vi "Process.vi"(11 "Message Queues out":T1) -> ()   [LabVIEW 2024]
doc: "This UI handle all the data process including data acquisition and calculations"
uses:
  Message Queue/All Message Queues.ctl
  Message Queue/Message Cluster.ctl
  controls/GlobalData.ctl
  controls/GlobalData.vi
  Message Queue/Enqueue Message (Single).vi
  Message Queue/Message Queue.lvlib
panel:
  out "Acquire Time":u32
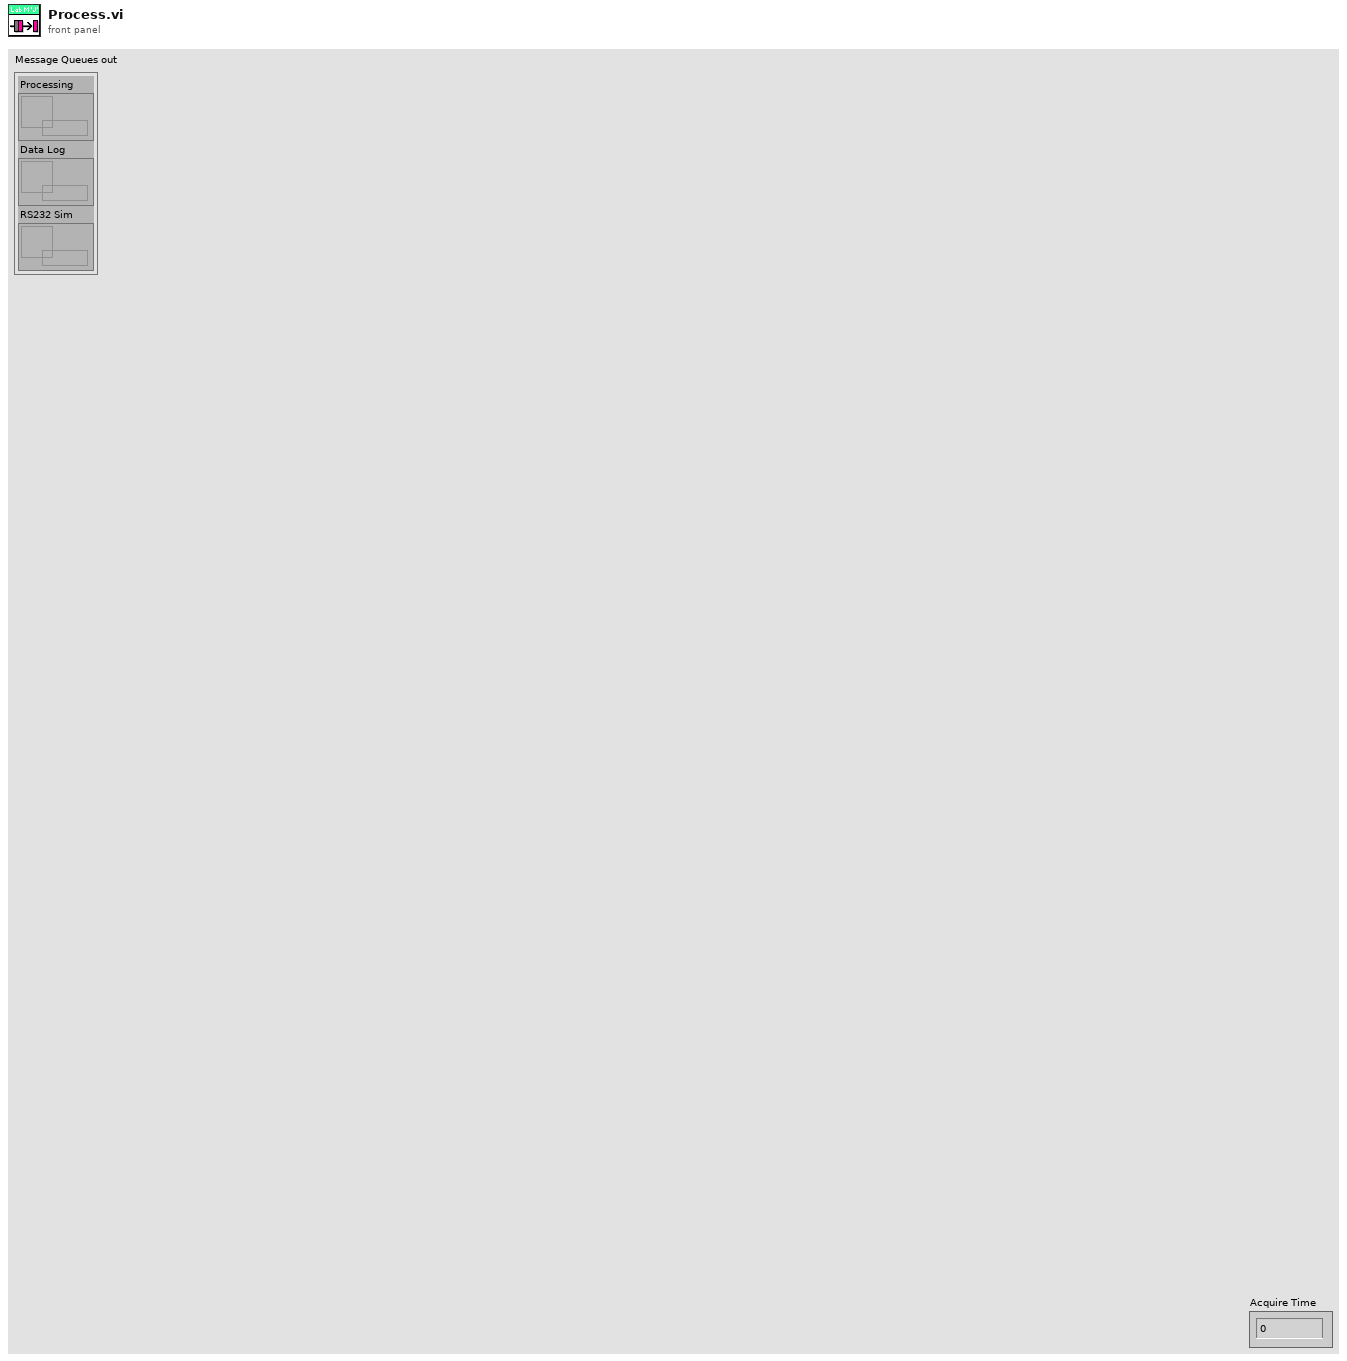
[diagram p1: front panel]
types:
  T1 = typedef "Message Queue.lvlib/All Message Queues.ctl" = cluster{"Processing":refnum<queue>, "Data Log":refnum<queue>, "RS232 Sim":refnum<queue>}
  T2 = typedef "GlobalData.ctl" = cluster{"Measurements":cluster{"Measurement Graphs":refnum<vi>, "Pressure":refnum<vi>, "Temperature":refnum<vi>, "Salinity":refnum<vi>, "Weight":refnum<vi>, "Pressure Raw":refnum<vi>, "Temperature Raw":refnum<vi>, "Salinity Raw":refnum<vi>, "Weight Raw":refnum<vi>, "Measurement Statstics":refnum<vi>, "Time Array":refnum<vi>}, "Settings":cluster{"Sampling Settings":refnum<vi>, "General Settings":refnum<vi>, "Disable Sensor Reading":refnum<vi>, "Units Settings":refnum<vi>, "Channels Settings":refnum<vi>, "Weight Port Settings":refnum<vi>}, "Calibration Data":cluster{"Pressure Cal":refnum<vi>, "Temperature Cal":refnum<vi>, "Salinity Cal":refnum<vi>, "Weight Cal":refnum<vi>}, "UI":cluster{"Generate Report":refnum<vi>}}
  T3 = cluster{"Pressure":dbl[], "Temperature":dbl[], "Salinity":dbl[], "Weight":dbl[]}
  T4 = cluster{"Measurement Statstics":bool, "Logging Type":enum16{"Disable Log", "TDMS", "CSV"}}
  T5 = cluster{"Reading Time (ms)":u64, "Graph Time ":u16}
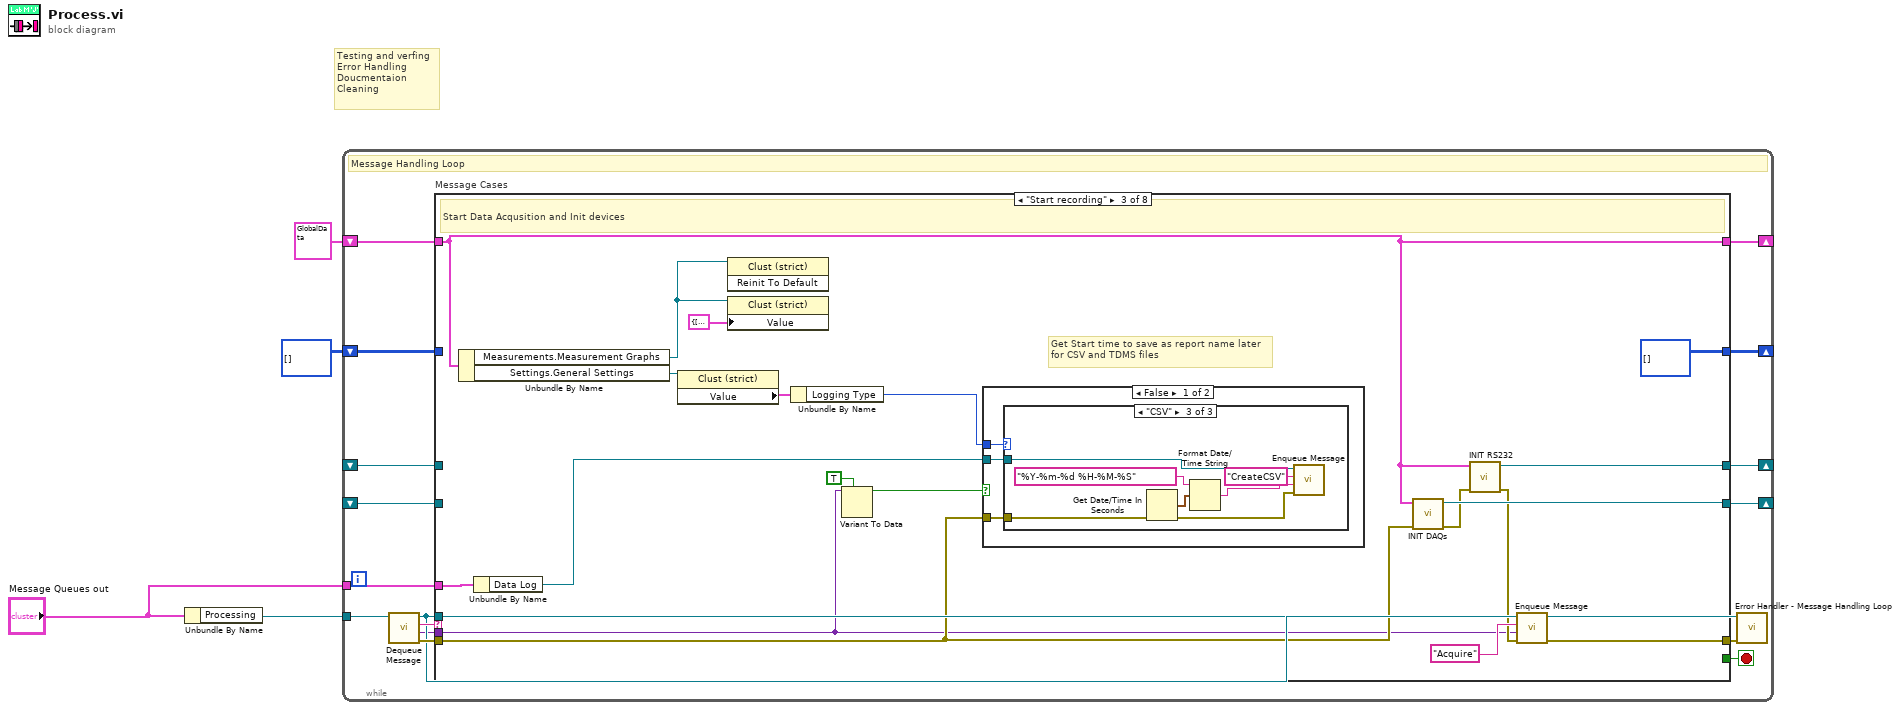
[diagram p0: block diagram]
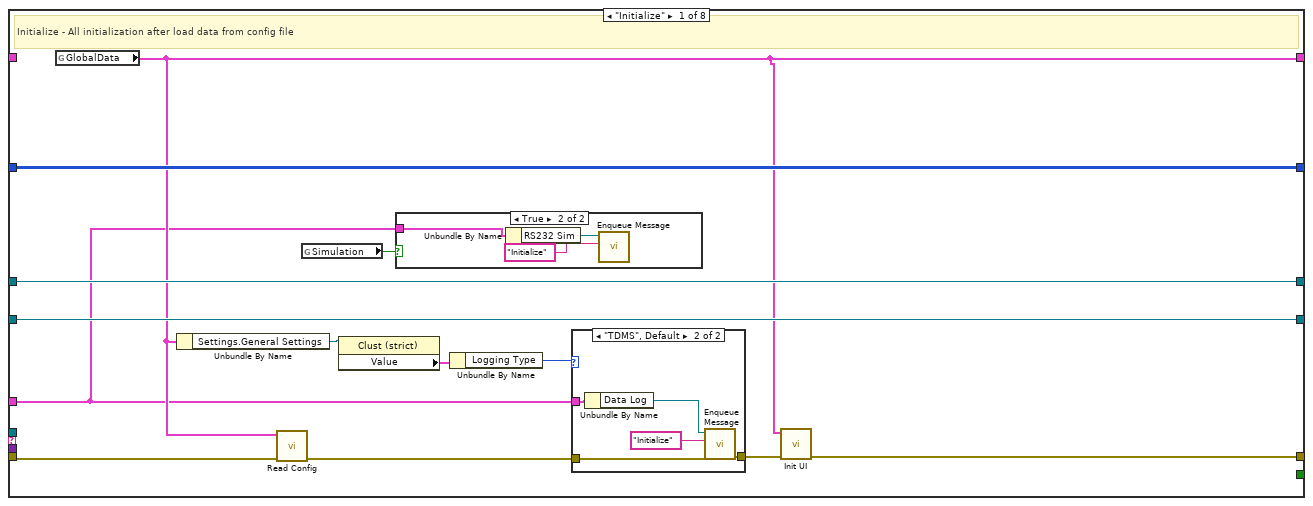
[diagram p2: hidden frame]
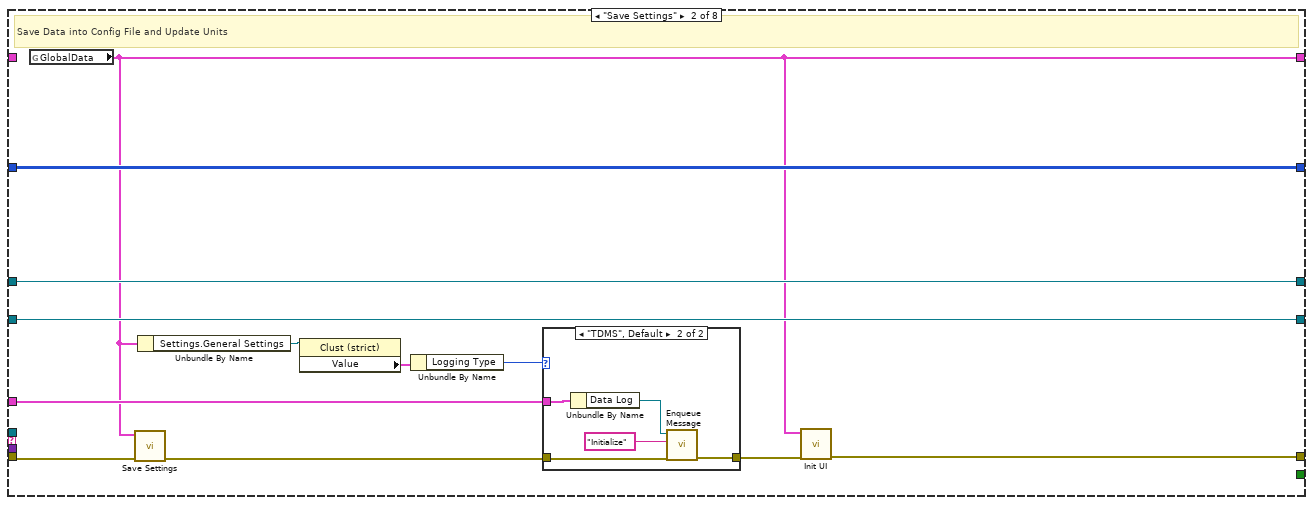
[diagram p5: hidden frame]
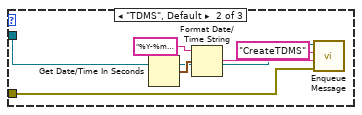
[diagram p8: hidden frame]
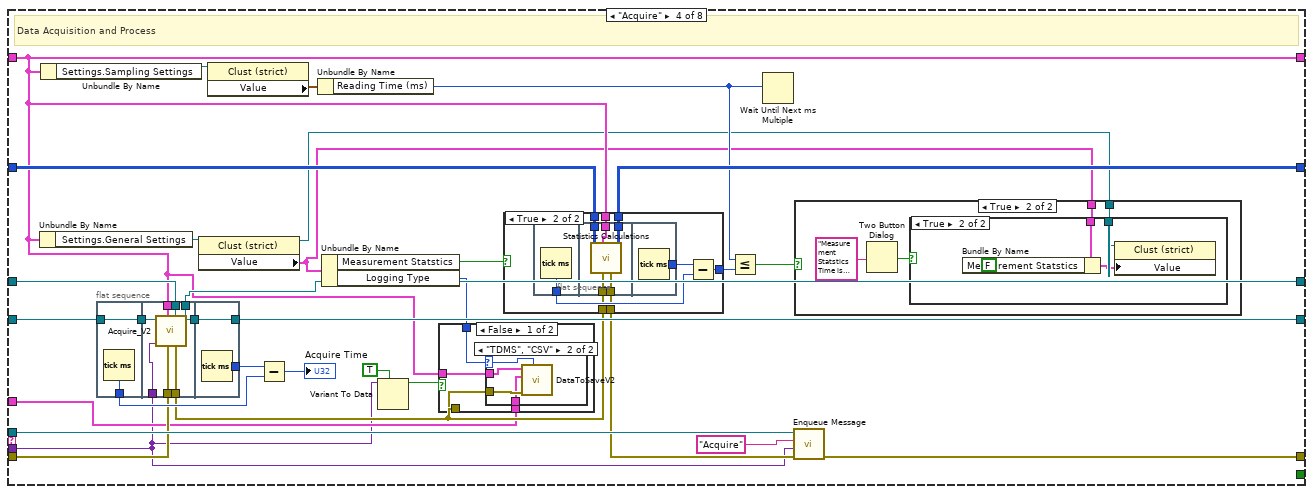
[diagram p10: hidden frame]
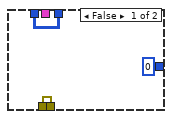
[diagram p15: hidden frame]
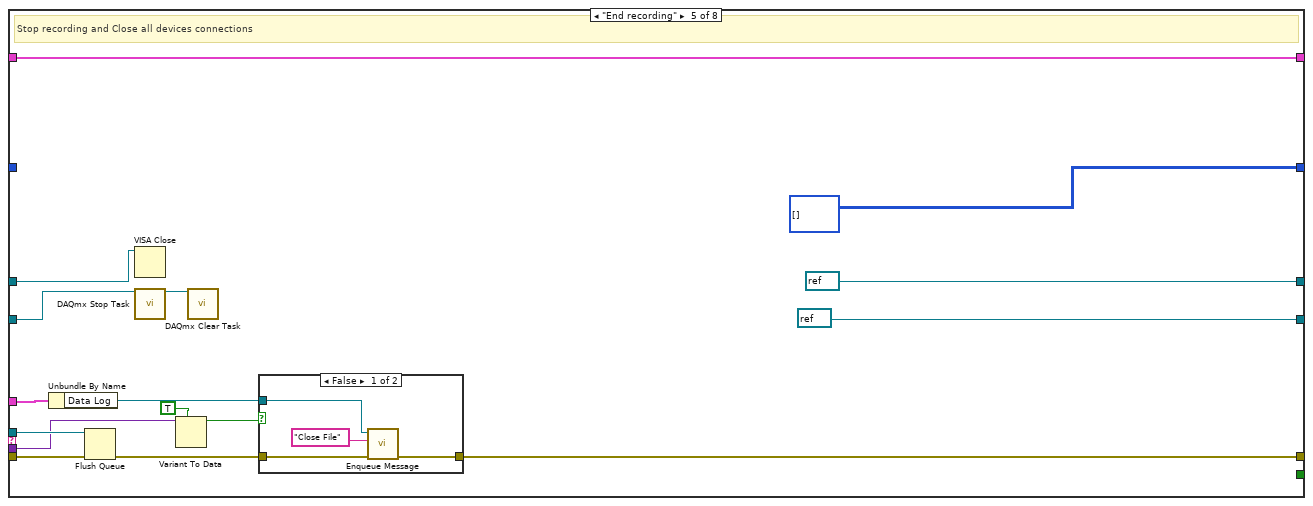
[diagram p16: hidden frame]
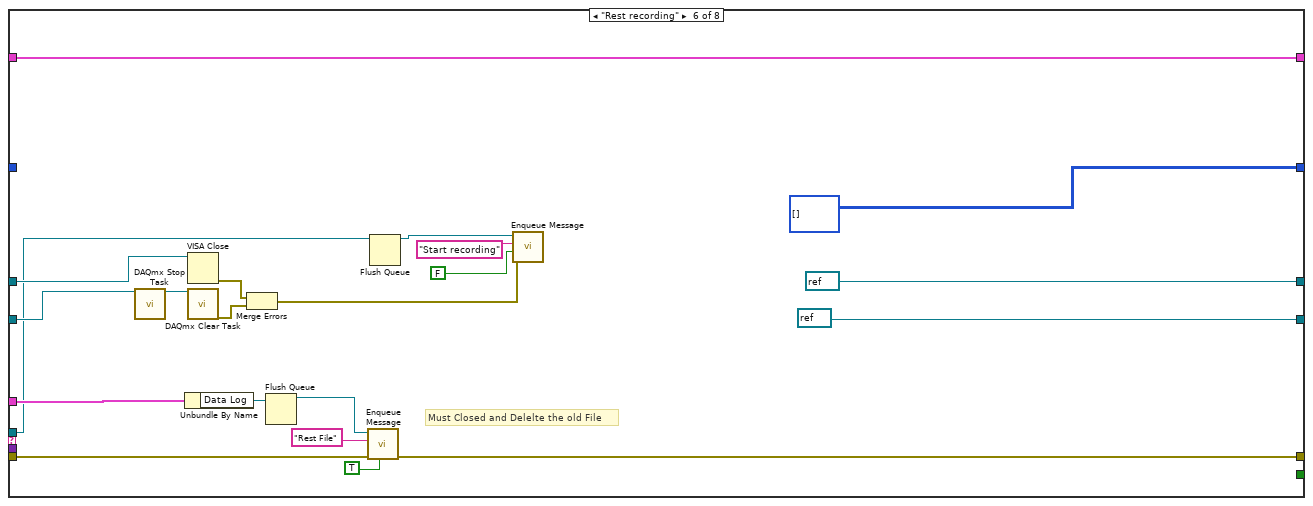
[diagram p18: hidden frame]
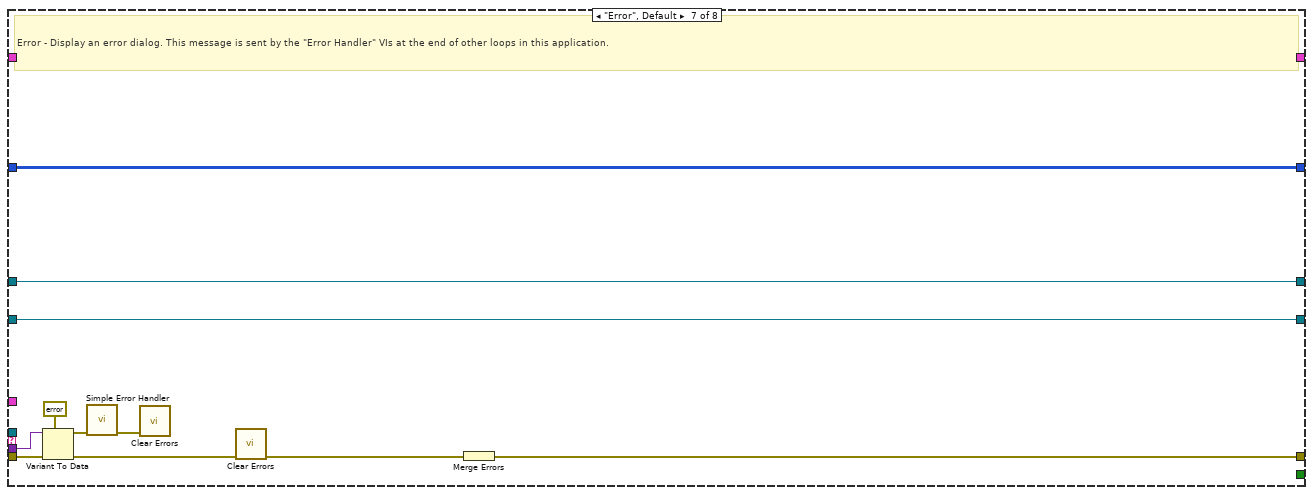
[diagram p19: hidden frame]
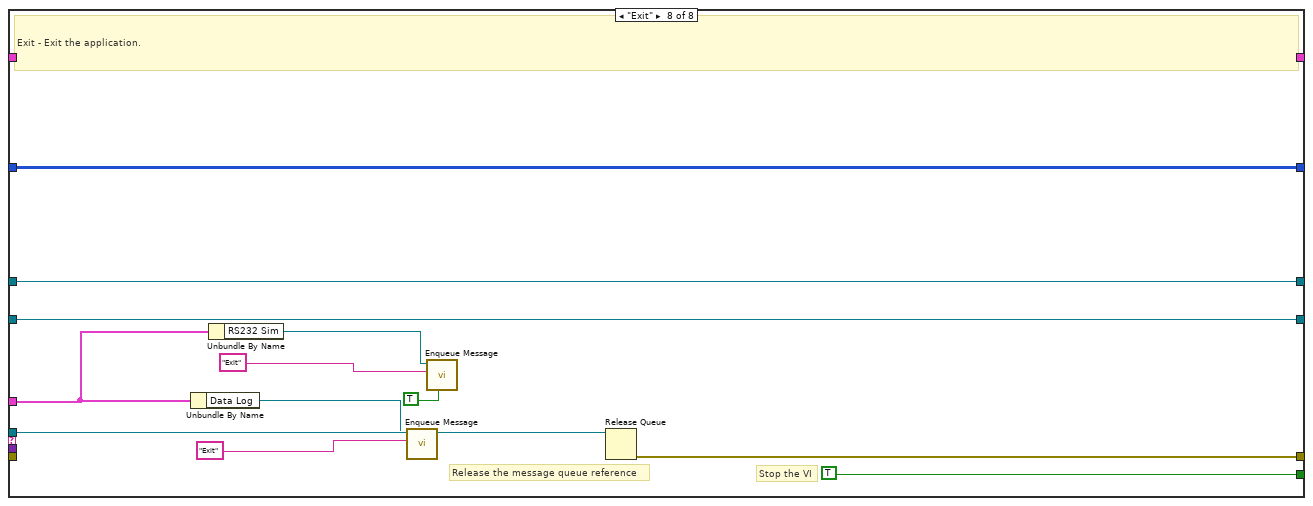
[diagram p20: hidden frame]
diagram:
  # "Testing and verfing\nError Handling \nDoucmentaion\nCleaning"
  n1 = Unbundle By Name("Message Queues out") -> ("Processing"=w4:refnum<queue>)
  n2 = while {
    tunnel: w4 -> [w15]
    shift-right: [w19] -> _
    shift-left: T2 {"Measurements"={"Measurement Graphs"=refnum, "Pressure"=refnum, "Temperature"=refnum, "Salinity"=refnum, "Weight"=refnum, "Pressure Raw"=refnum, "Temperature Raw"=refnum, "Salinity Raw"=refnum, "Weight Raw"=refnum, "Measurement Statstics"=refnum, "Time Array"=refnum}, "Settings"={"Sampling Settings"=refnum, "General Settings"=refnum, "Disable Sensor Reading"=refnum, "Units Settings"=refnum, "Channels Settings"=refnum, "Weight Port Settings"=refnum}, "Calibration Data"={"Pressure Cal"=refnum, "Temperature Cal"=refnum, "Salinity Cal"=refnum, "Weight Cal"=refnum}, "UI"={"Generate Report"=refnum}} ("GlobalData") -> [w20]
    shift-right: [w12] -> _
    shift-left: _ -> [w11]
    shift-right: [w9] -> _
    shift-left: i32[][] [] -> [w10]
    shift-right: [w7] -> _
    shift-left: _ -> [w6]
    tunnel: "Message Queues out" -> [w5]
    stop <- w18 stop-if-true
    # "Message Handling Loop"
    n3 = call "Dequeue Message.vi"("Message Queue"=w15) -> ("error out"=w17:errorcluster, "Message Data"=w8:variant, "Message"=w16:string, "dup Message Queue"=w14:refnum<queue>)  [unwired: 7 in]
    n4 = case "Message Cases" shown="\"Start recording\"" w16 {
      tunnel: w14 -> [_ _ w76 w124 w179 w204 _ w239]
      tunnel: w17 -> [w29 w49 w69 w105 w181 w206 w226 _]
      tunnel: [w30 w51 w78 w123 w180 w205 w221 w231] -> w13
      tunnel: w20 -> [_ _ w64 w102 w188 w214 w225 w238]
      tunnel: [w26 w44 w64 w102 w188 w214 w225 w238] -> w19
      tunnel: [_ _ _ _ _ _ _ TRUE] -> w18
      tunnel: [w33 w54 w80 w126 refnum<k21> refnum ("Pressure") refnum<k21> refnum ("Pressure") w220 w236] -> w12
      tunnel: w11 -> [w33 w54 _ w127 w186 w212 w220 w236]
      tunnel: w10 -> [w32 w53 _ w116 _ _ w219 w235]
      tunnel: [w32 w53 i32[][] [] ("Time Array") w115 i32[][] [] ("Time Array") i32[][] [] ("Time Array") w219 w235] -> w9
      tunnel: w8 -> [_ _ w62 w98 w174 _ w224 _]
      tunnel: [w31 w52 w74 w106 refnum<visa-resource-name> refnum ("Weight Port") refnum<visa-resource-name> refnum ("Weight Port") w218 w234] -> w7
      tunnel: w6 -> [w31 w52 _ w107 w184 w210 w218 w234]
      tunnel: w5 -> [w21 w50 w68 w101 w182 w207 _ w228]
      frame "Initialize" {
        # "Initialize - All initialization after load data from config file"
        n5 = global read "GlobalData.vi" "GlobalData"() -> (w26:T2)
        n6 = Unbundle By Name(w26) -> ("Settings.General Settings"=w25:refnum<vi>)
        n7 = call "Read Config.vi"("error in (no error)"=w29, "GlobalData"=w26) -> ("error out"=w28:errorcluster)  [unwired: 9 in]
        n8 = global read "GlobalData.vi" "Simulation"() -> (w22:bool)
        n9 = property class="Clust (strict)"(reference=w25) -> ("Value"=w24:T4)  [unwired: 1 in, 2 out]
        n10 = case shown="True" w22 {
          tunnel: w21 -> [_ w34]
          frame False {
          }
          frame True {
            n11 = Unbundle By Name(w34) -> ("RS232 Sim"=w36:refnum<queue>)
            n12 = call-poly "Enqueue Message.vi"("Message"="Initialize", "Message Queue"=w36) -> ()  [unwired: 8 in, 2 out]
          }
        }
        n13 = Unbundle By Name(w24) -> ("Logging Type"=w23:enum16{"Disable Log", "TDMS", "CSV"})
        n14 = case shown="\"TDMS\", Default" w23 {
          tunnel: w21 -> [_ w42]
          tunnel: w28 -> [w37 w39]
          tunnel: [w37 w38] -> w27
          frame "Disable Log" {
          }
          frame "TDMS", Default {
            n15 = Unbundle By Name(w42) -> ("Data Log"=w40:refnum<queue>)
            n16 = call-poly "Enqueue Message.vi"("error in (no error)"=w39, "Message"="Initialize", "Message Queue"=w40) -> ("error out"=w38:errorcluster)  [unwired: 7 in, 1 out]
          }
        }
        n17 = call "Init UI.vi"("error in (no error)"=w27, "GlobalData"=w26) -> ("error out"=w30:errorcluster)  [unwired: 9 in]
      }
      frame "Save Settings" {
        # "Save Data into Config File and Update Units"
        n18 = global read "GlobalData.vi" "GlobalData"() -> (w44:T2)
        n19 = call "Save Settings.vi"("error in (no error)"=w49, "GlobalData"=w44) -> ("error out"=w48:errorcluster)  [unwired: 9 in]
        n20 = Unbundle By Name(w44) -> ("Settings.General Settings"=w45:refnum<vi>)
        n21 = property class="Clust (strict)"(reference=w45) -> ("Value"=w46:T4)  [unwired: 1 in, 2 out]
        n22 = Unbundle By Name(w46) -> ("Logging Type"=w43:enum16{"Disable Log", "TDMS", "CSV"})
        n23 = case shown="\"TDMS\", Default" w43 {
          tunnel: w50 -> [_ w58]
          tunnel: w48 -> [w55 w57]
          tunnel: [w55 w56] -> w47
          frame "Disable Log" {
          }
          frame "TDMS", Default {
            n24 = Unbundle By Name(w58) -> ("Data Log"=w59:refnum<queue>)
            n25 = call-poly "Enqueue Message.vi"("error in (no error)"=w57, "Message"="Initialize", "Message Queue"=w59) -> ("error out"=w56:errorcluster)  [unwired: 7 in, 1 out]
          }
        }
        n26 = call "Init UI.vi"("error in (no error)"=w47, "GlobalData"=w44) -> ("error out"=w51:errorcluster)  [unwired: 9 in]
      }
      frame "Start recording" {
        # "Get Start time to save as report name later\nfor CSV and TDMS files"
        # "Start Data Acqusition and Init devices"
        n27 = Unbundle By Name(w64) -> ("Measurements.Measurement Graphs"=w66:refnum<vi>, "Settings.General Settings"=w71:refnum<vi>)
        n28 = Unbundle By Name(w68) -> ("Data Log"=w67:refnum<queue>)
        n29 = property class="Clust (strict)"(reference=w71) -> ("Value"=w72:T4)  [unwired: 1 in, 2 out]
        n30 = invoke class="Clust (strict)" method="Reinit To Default"(reference=w66) -> ()  [unwired: 2 in, 3 out]
        n31 = property class="Clust (strict)"(reference=w66, "Value"=T3 {"Pressure"=[], "Temperature"=[], "Salinity"=[], "Weight"=[]}) -> ()  [unwired: 1 in, 2 out]
        n32 = Unbundle By Name(w72) -> ("Logging Type"=w70:enum16{"Disable Log", "TDMS", "CSV"})
        n33 = Variant To Data(type=TRUE ("Calibration"), Variant=w62) -> (data=w61:bool)  [unwired: 1 in, 1 out]
        n34 = case shown="False" w61 {
          tunnel: w70 -> [w83 _]
          tunnel: w69 -> [w82 _]
          tunnel: w67 -> [w81 _]
          frame False {
            n35 = case shown="\"CSV\"" w83 {
              tunnel: w82 -> [_ w88 w94]
              tunnel: w81 -> [_ w85 w90]
              frame "Disable Log" {
              }
              frame "TDMS", Default {
                n36 = Get Date/Time In Seconds() -> (seconds since 1Jan1904=w87:timestamp)
                n37 = Format Date/Time String(time format string (%c)="%Y-%m-%d %H-%M-%S", seconds (now)=w87) -> (date/time string=w86:string)  [unwired: 1 in]
                n38 = call-poly "Enqueue Message.vi"("error in (no error)"=w88, "Message Data"=w86, "Message"="CreateTDMS", "Message Queue"=w85) -> ()  [unwired: 6 in, 2 out]
              }
              frame "CSV" {
                n39 = Get Date/Time In Seconds() -> (seconds since 1Jan1904=w93:timestamp)
                n40 = Format Date/Time String(time format string (%c)="%Y-%m-%d %H-%M-%S", seconds (now)=w93) -> (date/time string=w91:string)  [unwired: 1 in]
                n41 = call-poly "Enqueue Message.vi"("error in (no error)"=w94, "Message Data"=w91, "Message"="CreateCSV", "Message Queue"=w90) -> ()  [unwired: 6 in, 2 out]
              }
            }
          }
          frame True {
          }
        }
        n42 = call "INIT DAQs.vi"("error in (no error)"=w69, "GlobalData"=w64) -> ("error out"=w75:errorcluster, "Pressure"=w80:refnum<k21>)  [unwired: 8 in]
        n43 = call "INIT RS232.vi"("error in (no error)"=w75, "GlobalData"=w64) -> ("error out"=w73:errorcluster, "Weight Port"=w74:refnum<visa-resource-name>)  [unwired: 8 in]
        n44 = call-poly "Enqueue Message.vi"("error in (no error)"=w73, "Message Data"=w62, "Message"="Acquire", "Message Queue"=w76) -> ("error out"=w78:errorcluster)  [unwired: 6 in, 1 out]
      }
      frame "Acquire" {
        # "Data Acquisition and Process"
        n45 = Unbundle By Name(w102) -> ("Settings.General Settings"=w114:refnum<vi>)
        n46 = Unbundle By Name(w102) -> ("Settings.Sampling Settings"=w122:refnum<vi>)
        n47 = flat-sequence {
          tunnel: w127 -> [w163]
          tunnel: [w163] -> w120
          tunnel: [w162] -> w117
          tunnel: w105 -> [w169]
          tunnel: [w168] -> w104
          tunnel: w120 -> [w171]
          tunnel: [w170] -> w119
          tunnel: w98 -> [w167]
          tunnel: w102 -> [w166]
          tunnel: w107 -> [w165]
          tunnel: [w164] -> w106
          tunnel: [w173] -> w126
          tunnel: w119 -> [w173]
          tunnel: [w172] -> w118
          frame #0 {
            n48 = Tick Count (ms)() -> (millisecond timer value=w162:u32)
          }
          frame #1 {
            n49 = call "Acquire_V2.vi"("Weight Port"=w165, "error in"=w169, "GlobalData"=w166, "Calibration"=w167, "Pressure"=w171) -> ("Weight Port"=w164:refnum<visa-resource-name>, "Pressure"=w170:refnum<k21>, "error out"=w168:errorcluster)  [unwired: 4 in]
          }
          frame #2 {
            n50 = Tick Count (ms)() -> (millisecond timer value=w172:u32)
          }
        }
        n51 = property class="Clust (strict)"(reference=w114) -> (reference out=w100:refnum<vi>, "Value"=w99:T4)  [unwired: 1 in, 1 out]
        n52 = property class="Clust (strict)"(reference=w122) -> ("Value"=w121:T5)  [unwired: 1 in, 2 out]
        n53 = Subtract(x=w118, y=w117) -> (x-y=→"Acquire Time":u32)
        n54 = Unbundle By Name(w121) -> ("Reading Time (ms)"=w109:u64)
        n55 = Unbundle By Name(w99) -> ("Measurement Statstics"=w113:bool, "Logging Type"=w103:enum16{"Disable Log", "TDMS", "CSV"})
        n56 = Variant To Data(type=TRUE ("Calibration"), Variant=w98) -> (data=w96:bool)  [unwired: 1 in, 1 out]
        n57 = case shown="False" w96 {
          tunnel: w104 -> [w131 _]
          tunnel: w103 -> [w130 _]
          tunnel: w102 -> [w129 _]
          tunnel: w101 -> [w128 _]
          frame False {
            n58 = case shown="\"TDMS\", \"CSV\"" w130 {
              selector: w130 -> [_ w134]
              tunnel: w131 -> [_ w135]
              tunnel: w129 -> [_ w133]
              tunnel: w128 -> [_ w132]
              frame "Disable Log", Default {
              }
              frame "TDMS", "CSV" {
                n59 = call "DataToSaveV2.vi"("Logging Type"=w134, "error in (no error)"=w135, "Message Queues out"=w132, "GlobalData"=w133) -> ()  [unwired: 7 in, 1 out]
              }
            }
          }
          frame True {
          }
        }
        n60 = case shown="True" w113 {
          tunnel: w116 -> [w146 w152]
          tunnel: [w146 w151] -> w115
          tunnel: w104 -> [w145 w150]
          tunnel: [w145 w149] -> w112
          tunnel: [u32 0 w148] -> w110
          tunnel: w102 -> [_ w147]
          frame False {
          }
          frame True {
            n61 = flat-sequence {
              tunnel: [w155] -> w154
              tunnel: w152 -> [w160]
              tunnel: [w159] -> w151
              tunnel: w150 -> [w158]
              tunnel: [w157] -> w149
              tunnel: w147 -> [w156]
              tunnel: [w161] -> w153
              frame #0 {
                n62 = Tick Count (ms)() -> (millisecond timer value=w155:u32)
              }
              frame #1 {
                n63 = call "Statistics Calculations.vi"("error in"=w158, "GlobalData"=w156, "Time Array"=w160) -> ("Time Array"=w159:i32[][], "error out"=w157:errorcluster)  [unwired: 7 in]
              }
              frame #2 {
                n64 = Tick Count (ms)() -> (millisecond timer value=w161:u32)
              }
            }
            n65 = Subtract(x=w153, y=w154) -> (x-y=w148:u32)
          }
        }
        n66 = Less Or Equal?(x=w109, y=w110) -> (x <= y?=w108:bool)
        n67 = Wait Until Next ms Multiple(millisecond multiple=w109) -> ()  [unwired: 1 out]
        n68 = call-poly "Enqueue Message.vi"("error in (no error)"=w112, "Message Data"=w98, "Message"="Acquire", "Message Queue"=w124) -> ("error out"=w123:errorcluster)  [unwired: 6 in, 1 out]
        n69 = case shown="True" w108 {
          tunnel: w100 -> [_ w137]
          tunnel: w99 -> [_ w136]
          frame False {
          }
          frame True {
            n70 = Two Button Dialog(message="Measurement Statstics Time is bigger than Sampling time , please disable Measurement Statstics or dicrease sampling time ! , Do you Want to Disable Measurement Statstics") -> (T button?=w138:bool)  [unwired: 2 in]
            n71 = case shown="True" w138 {
              tunnel: w137 -> [_ w143]
              tunnel: w136 -> [_ w142]
              frame False {
              }
              frame True {
                n72 = Bundle By Name(cluster=w142, "Measurement Statstics"=FALSE) -> (w140:T4)
                n73 = property class="Clust (strict)"(reference=w143, "Value"=w140) -> ()  [unwired: 1 in, 2 out]
              }
            }
          }
        }
      }
      frame "End recording" {
        # "Stop recording and Close all devices connections"
        n74 = Unbundle By Name(w182) -> ("Data Log"=w178:refnum<queue>)
        n75 = Flush Queue(queue=w179) -> ()  [unwired: 1 in, 3 out]
        n76 = VISA Close(VISA resource name=w184) -> ()  [unwired: 1 in, 1 out]
        n77 = call <vilib>:"DAQmx Stop Task.vi"("task/channels in"=w186) -> ("task out"=w187:refnum<k21>)  [unwired: 13 in, 1 out]
        n78 = Variant To Data(type=TRUE ("Calibration"), Variant=w174) -> (data=w175:bool)  [unwired: 1 in, 1 out]
        n79 = call <vilib>:"DAQmx Clear Task.vi"("task in"=w187) -> ()  [unwired: 14 in, 1 out]
        n80 = case shown="False" w175 {
          tunnel: w181 -> [w191 w193]
          tunnel: [w190 w193] -> w180
          tunnel: w178 -> [w189 _]
          frame False {
            n81 = call-poly "Enqueue Message.vi"("error in (no error)"=w191, "Message"="Close File", "Message Queue"=w189) -> ("error out"=w190:errorcluster)  [unwired: 7 in, 1 out]
          }
          frame True {
          }
        }
      }
      frame "Rest recording" {
        # "Must Closed and Delelte the old File"
        n82 = call <vilib>:"DAQmx Stop Task.vi"("task/channels in"=w212) -> ("task out"=w213:refnum<k21>)  [unwired: 13 in, 1 out]
        n83 = Unbundle By Name(w207) -> ("Data Log"=w195:refnum<queue>)
        n84 = VISA Close(VISA resource name=w210) -> (error out=w199:errorcluster)  [unwired: 1 in]
        n85 = call <vilib>:"DAQmx Clear Task.vi"("task in"=w213) -> ("error out"=w200:errorcluster)  [unwired: 14 in]
        n86 = Merge Errors(w199, w200) -> (w198:errorcluster)
        n87 = Flush Queue(queue=w195) -> (queue out=w194:refnum<queue>)  [unwired: 1 in, 2 out]
        n88 = call-poly "Enqueue Message.vi"("Priority Message? (F)"=TRUE, "error in (no error)"=w206, "Message"="Rest File", "Message Queue"=w194) -> ("error out"=w205:errorcluster)  [unwired: 6 in, 1 out]
        n89 = Flush Queue(queue=w204) -> (queue out=w203:refnum<queue>)  [unwired: 1 in, 2 out]
        n90 = call-poly "Enqueue Message.vi"("error in (no error)"=w198, "Message Data"=FALSE ("Discard?"), "Message"="Start recording", "Message Queue"=w203) -> ()  [unwired: 6 in, 2 out]
      }
      frame "Error", Default {
        # "Error - Display an error dialog. This message is sent by the \"Error Handler\" VIs at the end of other loops in this application."
        n91 = Variant To Data(error in=w226, type=errorcluster {"status"=FALSE, "code"=0, "source"=""} ("error constant"), Variant=w224) -> (data=w222:errorcluster, error out=w216:errorcluster)
        n92 = call <vilib>:"Simple Error Handler.vi"("error in (no error)"=w222) -> ("error out"=w217:errorcluster)  [unwired: 4 in, 4 out]
        n93 = call <vilib>:"Clear Errors.vi"("error in (no error)"=w217) -> ()  [unwired: 5 in, 2 out]
        n94 = call <vilib>:"Clear Errors.vi"("error in (no error)"=w216) -> ("error out"=w215:errorcluster)  [unwired: 5 in, 1 out]
        n95 = Merge Errors(w215) -> (w221:errorcluster)
      }
      frame "Exit" {
        # "Stop the VI"
        # "Release the message queue reference"
        # "Exit - Exit the application."
        n96 = Unbundle By Name(w228) -> ("Data Log"=w232:refnum<queue>)
        n97 = Unbundle By Name(w228) -> ("RS232 Sim"=w230:refnum<queue>)
        n98 = call-poly "Enqueue Message.vi"("Message"="Exit", "Message Queue"=w232) -> ()  [unwired: 8 in, 2 out]
        n99 = call-poly "Enqueue Message.vi"("Priority Message? (F)"=TRUE, "Message"="Exit", "Message Queue"=w230) -> ()  [unwired: 7 in, 2 out]
        n100 = Release Queue(queue=w239) -> (error out=w231:errorcluster)  [unwired: 2 in, 2 out]
      }
    }
    n101 = call "Error Handler - Message Handling Loop.vi"("error in (no error)"=w13, "Message Queue"=w14) -> ()  [unwired: 8 in, 2 out]
  }
